vi "convertWavelengthToRamanShift.vi"(10 "wavelengths":dbl[](array[numeric]), 11 "excitationWavelength":dbl) -> (3 "Array":dbl[](array[numeric]))   [LabVIEW 2020, in "horiba.lvlib" / "CCD.lvclass"]
uses:
  CCD.lvclass
panel:
  # "Connector Pane"
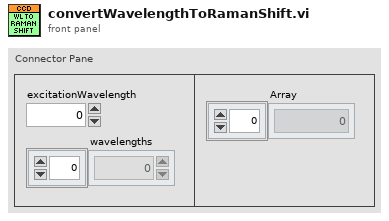
[diagram p1: front panel]
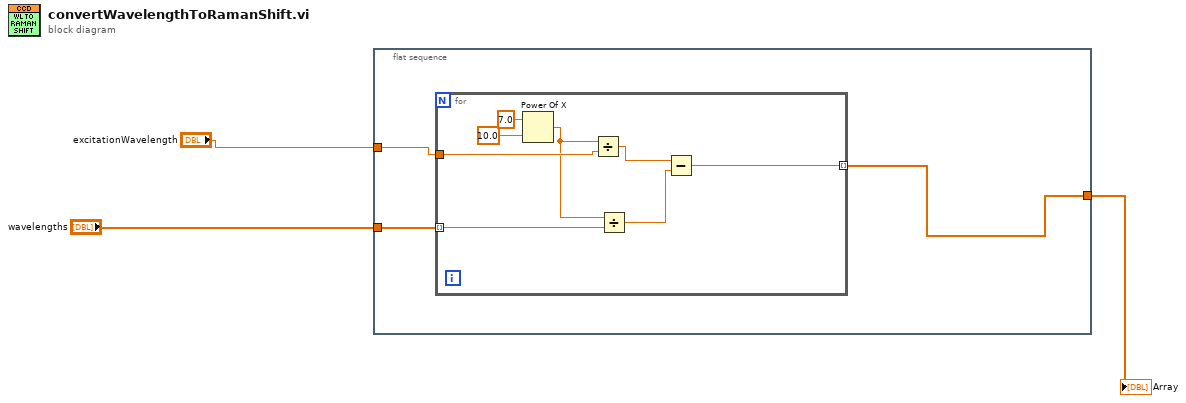
[diagram p0: block diagram]
diagram:
  n1 = flat-sequence {
    tunnel: "excitationWavelength" -> [w5]
    tunnel: "wavelengths" -> [w6]
    tunnel: [w4] -> w3
    frame #0 {
      n2 = for {
        tunnel: w6 -> [w9] mode=indexing
        tunnel: w5 -> [w12]
        tunnel: [w7] -> w4 mode=indexing
        n3 = Power Of X(1:10.0 ("y"), 2:7.0 ("x")) -> (0:w10:dbl)
        n4 = Divide(x=w10, y=w12) -> (x/y=w11:dbl)
        n5 = Divide(x=w10, y=w9) -> (x/y=w8:dbl)
        n6 = Subtract(x=w11, y=w8) -> (x-y=w7:dbl)
      }
    }
  }
  "Array" <- w3
